vi "AddValue.vi"(1 "Display State In":T2 caption="State", 2 "Data In":T1) -> (0 "Display State Out":T2 caption="State")   [LabVIEW 2011, in "VariantXControl__VP.xctl"]
uses:
  VariantXControl__VP.xctl
  VariantState.ctl
  Permissions.ctl
  TreeSettings.ctl
  VariantData.ctl
  VariantTree__VP.lvclass
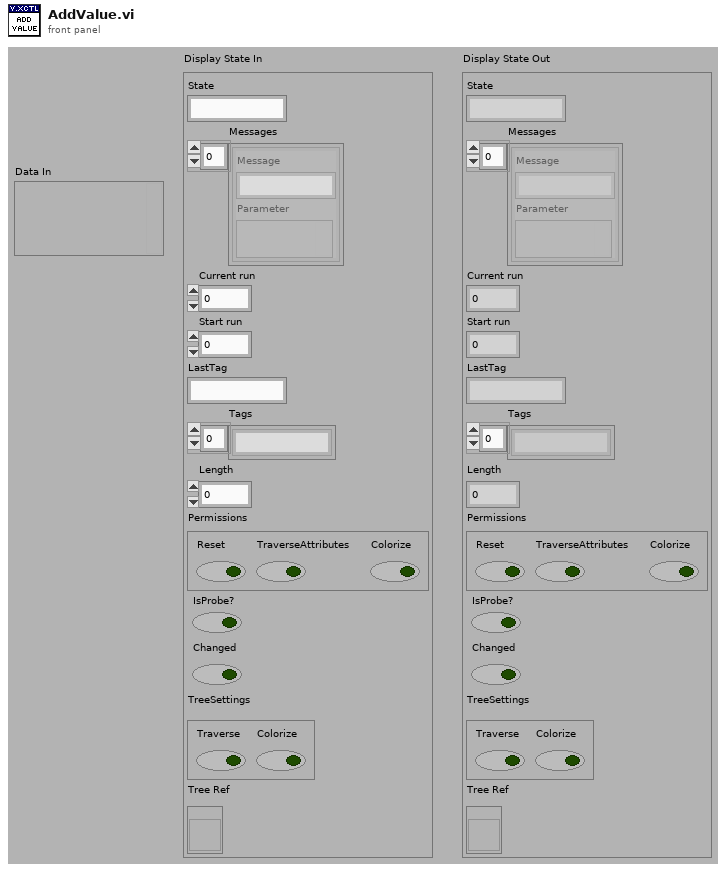
[diagram p1: front panel]
types:
  T1 = typedef "VariantXControl__VP.xctl/VariantData.ctl" = variant
  T2 = typedef "VariantXControl__VP.xctl/VariantState.ctl" = cluster{"State":string, "Messages":cluster{"Message":string, "Parameter":variant}[], "Current run":i32, "Start run":i32, "LastTag":string, "Tags":string[], "Length":i32, "Permissions":T3, "IsProbe?":bool, "Changed":bool, "TreeSettings":T4, "Tree Ref":refnum<vi>}
  T3 = typedef "VariantXControl__VP.xctl/Permissions.ctl" = cluster{"Reset":bool, "TraverseAttributes":bool, "Colorize":bool}
  T4 = typedef "VariantXControl__VP.xctl/TreeSettings.ctl" = cluster{"Traverse":bool, "Colorize":bool}
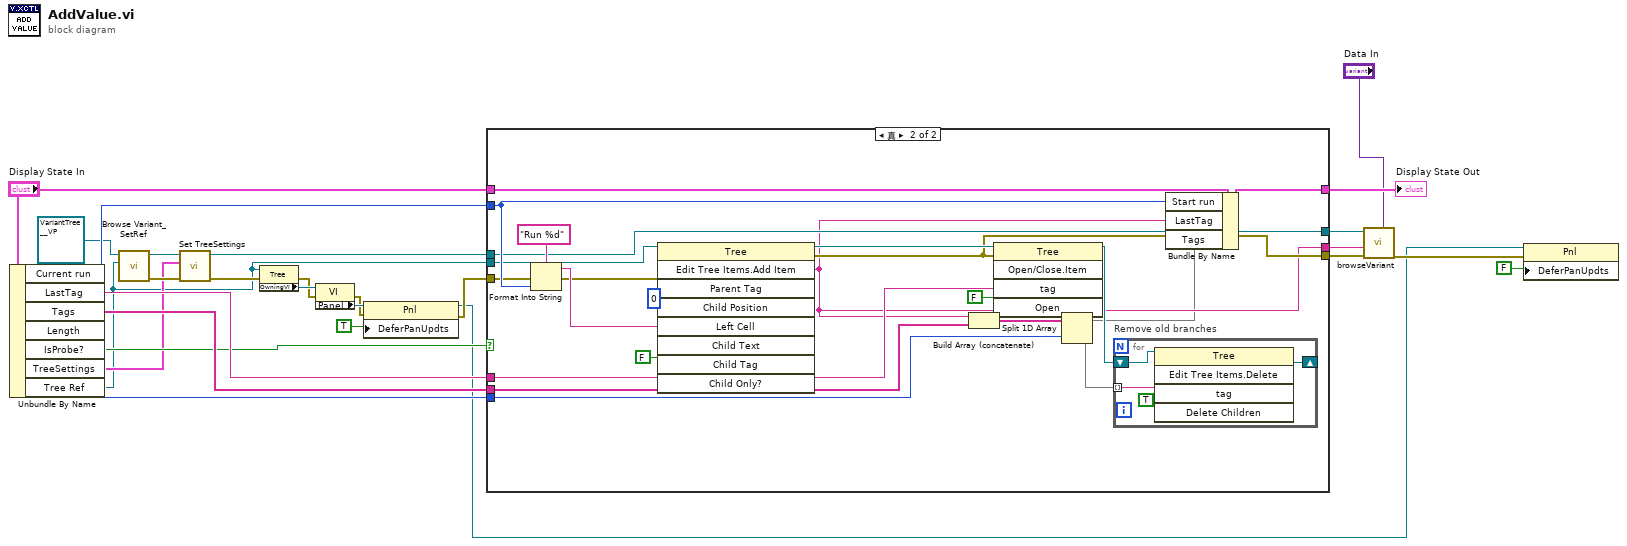
[diagram p0: block diagram]
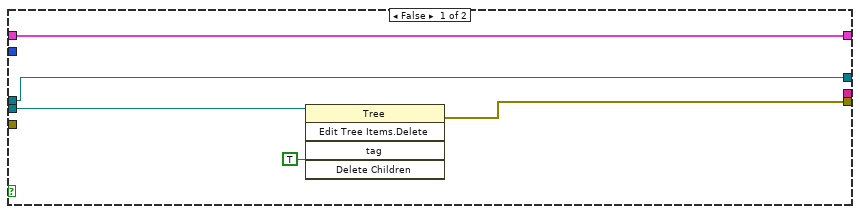
[diagram p2: hidden frame]
diagram:
  n1 = Unbundle By Name("Display State In") -> ("Current run"=w24:i32, "LastTag"=w21:string, "Tags"=w22:string[], "Length"=w23:i32, "IsProbe?"=w17:bool, "TreeSettings"=w4:T4, "Tree Ref"=w1:refnum<vi>)
  n2 = call "Browse Variant_SetRef.vi"("Tree Ref"=w1, "Dummy Class.lvclass in"=refnum<class "VariantTree__VP.lvclass"> refnum ("Dummy Class.lvclass")) -> ("error out"=w5:errorcluster, "Dummy Class.lvclass out"=w6:refnum<class "VariantTree__VP.lvclass">)  [unwired: 8 in]
  n3 = call-dynamic "Set TreeSettings.vi"("error in (no error)"=w5, "TreeSettings"=w4, "VariantTree.lvclass in"=w6) -> ("error out"=w2:errorcluster, "VariantTree.lvclass out"=w3:refnum<class "VariantTree__VP.lvclass">)  [unwired: 7 in]
  n4 = property class="Tree"(reference=w1, error in=w2) -> (error out=w15:errorcluster, "OwningVI"=w16:refnum<vi>)  [unwired: 1 out]
  n5 = property class="VI"(reference=w16, error in=w15) -> (error out=w12:errorcluster, "Panel"=w14:refnum<vi>)  [unwired: 1 out]
  n6 = property class="Pnl"(reference=w14, error in=w12, "DeferPanUpdts"=TRUE ("Defer Panel Updates")) -> (reference out=w8:refnum<vi>, error out=w11:errorcluster)
  n7 = case shown="真" w17 {
    tunnel: [w32 w54] -> w27
    tunnel: "Display State In" -> [w32 w53]
    tunnel: w24 -> [_ w52]
    tunnel: w23 -> [_ w49]
    tunnel: w22 -> [_ w47]
    tunnel: w21 -> [_ w46]
    tunnel: [_ w34] -> w20
    tunnel: w3 -> [w31 w37]
    tunnel: [w31 w37] -> w19
    tunnel: [w28 w35] -> w18
    tunnel: w1 -> [w29 w40]
    tunnel: w11 -> [_ w38]
    frame False {
      n8 = invoke class="Tree" method="Edit Tree Items.Delete"(reference=w29, "Delete Children"=TRUE ("Delete Children?")) -> (error out=w28:errorcluster)  [unwired: 3 in, 4 out]
    }
    frame True {
      n9 = Format Into String(format string="Run %d" ("Left Cell String"), error in=w38, w52) -> (resulting string=w44:string, error out=w39:errorcluster)  [unwired: 1 in]
      n10 = invoke class="Tree" method="Edit Tree Items.Add Item"(reference=w40, error in=w39, "Child Position"=0, "Left Cell"=w44, "Child Only?"=FALSE) -> (reference out=w36:refnum<vi>, error out=w35:errorcluster, "Edit Tree Items:Add Item"=w34:string)  [unwired: 4 in, 6 out]
      n11 = Build Array (concatenate)(w34, w47) -> (w51:string[])
      n12 = invoke class="Tree" method="Open/Close.Item"(reference=w36, error in=w35, "tag"=w46, "Open"=FALSE ("Open?")) -> (reference out=w45:refnum<vi>)  [unwired: 1 in, 4 out]
      n13 = Split 1D Array(array=w51, index=w49) -> (first subarray=w33:string[], second subarray=w50:string[])
      n14 = for "Remove old branches" {
        tunnel: w50 -> [w57] mode=indexing
        shift-right: [w55] -> _
        shift-left: w45 -> [w56]
        n15 = invoke class="Tree" method="Edit Tree Items.Delete"(reference=w56, "tag"=w57, "Delete Children"=TRUE ("Delete Children?")) -> (reference out=w55:refnum<vi>)  [unwired: 2 in, 4 out]
      }
      n16 = Bundle By Name(cluster=w53, "Start run"=w52, "LastTag"=w34, "Tags"=w33) -> (w54:T2)
    }
  }
  "Display State Out" <- w27
  n17 = call-dynamic "browseVariant.vi"("Variant"="Data In", "error in (no error)"=w18, "ParentTag"=w20, "VariantProbe.lvclass in"=w19) -> ("error out"=w9:errorcluster)  [unwired: 4 in, 1 out]
  n18 = property class="Pnl"(reference=w8, error in=w9, "DeferPanUpdts"=FALSE ("Defer Panel Updates")) -> ()  [unwired: 2 out]
